vi "Load Sequence.vi"(8 "error in (no error)":errorcluster, 10 "Sequence Name":string, 11 "Sequencing Control in":refnum<class "Sequencing Control.lvclass">) -> (0 "error out":errorcluster, 3 "Sequencing Control out":refnum<class "Sequencing Control.lvclass">)   [LabVIEW 2023, in "VolatusSeqGUI.lvlib" / "Sequencing Control.lvclass"]
uses:
  Sequencing Control.lvclass
  Sequencing Control.lvclass/Sequencing Control.ctl
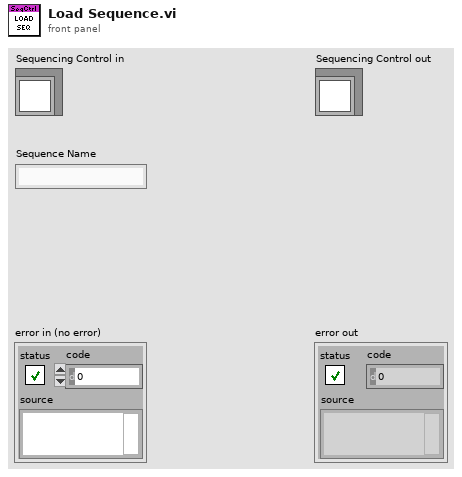
[diagram p1: front panel]
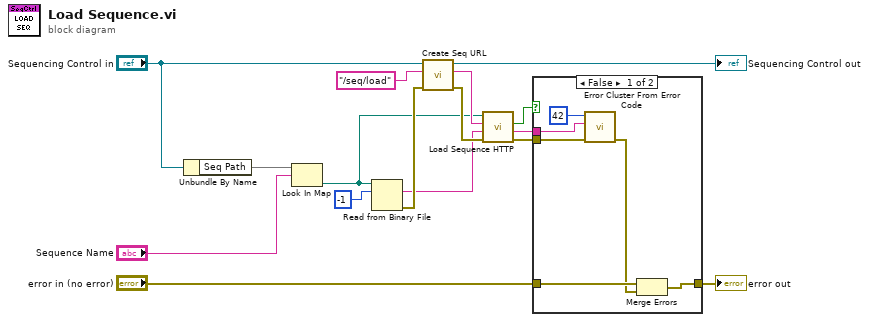
[diagram p0: block diagram]
diagram:
  n1 = Unbundle By Name("Sequencing Control in") -> ("Seq Path"=w14:map{string, path})
  n2 = Look In Map(map=w14, key="Sequence Name") -> (value=w1:path)  [unwired: 1 in, 1 out]
  n3 = Read from Binary File(10:-1 ("count (1)"), 11:w1) -> (0:w16:errorcluster, 2:w10:string)  [unwired: 4 in, 2 out]
  n4 = call "Create Seq URL.vi"("error in (no error)"=w16, "Path"="/seq/load", "Sequencing Control in"="Sequencing Control in") -> ("error out"=w15:errorcluster, "Request URL"=w2:string, "Sequencing Control out"=→"Sequencing Control out":refnum<class "Sequencing Control.lvclass">)  [unwired: 6 in]
  n5 = call "Load Sequence HTTP.vi"("error in (no error)"=w15, "VSEQ"=w10, "URL"=w2, "Path"=w1) -> ("error out"=w6:errorcluster, "Message"=w5:string, "Success"=w9:bool)  [unwired: 5 in]
  n6 = case shown="False" w9 {
    tunnel: [w17 w23] -> w8
    tunnel: "error in (no error)" -> [w19 w23]
    tunnel: w6 -> [w22 _]
    tunnel: w5 -> [w21 _]
    frame False {
      n7 = call <vilib>:"Error Cluster From Error Code.vi"("error in (no error)"=w22, "error message (\"\")"=w21, "error code (0)"=42) -> ("error out"=w18:errorcluster)  [unwired: 6 in]
      n8 = Merge Errors(w19, w18) -> (w17:errorcluster)
    }
    frame True {
    }
  }
  "error out" <- w8
